vi "VFD_Motor_Run.vi"(7 "PWM Frequency [Hz]":dbl=10000.0, 9 "Motor speed (%)":dbl=1.0 min=1.0 max=70.0) -> (3 "task out":refnum<k21>)   [LabVIEW 2021]
uses:
  Human_Labview/global_variables.vi
  <vilib>/DAQmx/create/channels.llb/DAQmx Create Channel (CO-Pulse Generation-Frequency).vi
  <vilib>/DAQmx/configure/timing.llb/DAQmx Timing (Implicit).vi
  <resource>/objmgr/daqmx.rc
panel:
  out "Actual Duty Cycle":dbl=0.01
  out "Actual Freq":dbl=200.0
  out "[PWM Duty Cycle %]\nMOTOR Speed Analog \nVoltage Control":dbl(slide)=1.0 scale=0.0..100.0
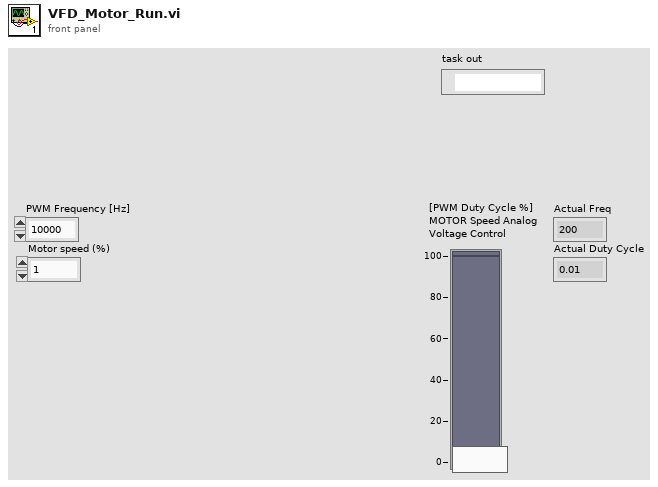
[diagram p1: front panel]
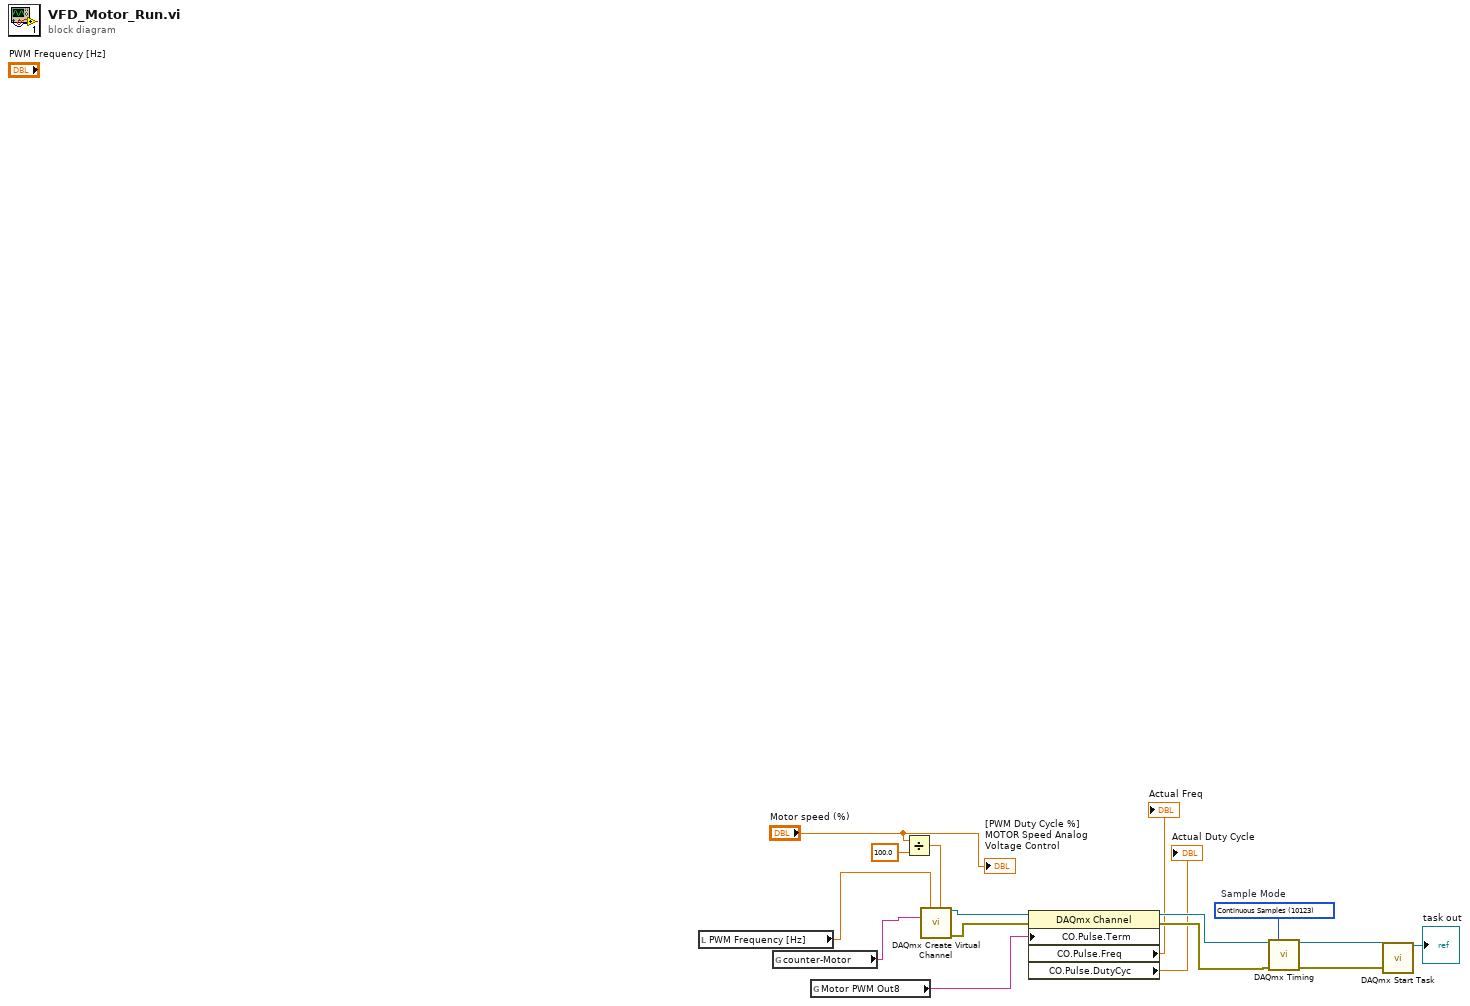
[diagram p0: block diagram]
diagram:
  w3 = 10123 items=["Finite Samples"=10178, "Continuous Samples"=10123, "Hardware Timed Single Point"=12522]  # Sample Mode
  n1 = local read "PWM Frequency [Hz]"() -> (w15:dbl)
  n2 = global read "global_variables.vi" "counter-Motor"() -> (w16:tag)
  n3 = global read "global_variables.vi" "Motor PWM Out8"() -> (w14:tag)
  n4 = Divide(x="Motor speed (%)", y=100.0) -> (x/y=w4:dbl)
  n5 = call-poly <vilib>:"DAQmx Create Virtual Channel.vi"("frequency"=w15, "duty cycle"=w4, "counter"=w16) -> ("task out"=w7:refnum<k21>, "error out"=w8:errorcluster)  [unwired: 11 in]
  n6 = property class="DAQmx Channel"(reference=w7, error in=w8, "CO.Pulse.Term"=w14) -> (reference out=w9:refnum<k21>, error out=w10:errorcluster, "CO.Pulse.Freq"=→"Actual Freq":dbl, "CO.Pulse.DutyCyc"=→"Actual Duty Cycle":dbl)
  n7 = call-poly <vilib>:"DAQmx Timing.vi"("task/channels in"=w9, "sample mode"=w3, "error in"=w10) -> ("task out"=w12:refnum<k21>, "error out"=w11:errorcluster)  [unwired: 11 in]
  n8 = call <vilib>:"DAQmx Start Task.vi"("task/channels in"=w12, "error in"=w11) -> ("task out"=→"task out":refnum<k21>)  [unwired: 12 in, 1 out]
  "[PWM Duty Cycle %]\nMOTOR Speed Analog \nVoltage Control" <- "Motor speed (%)"
